vi "Output_Curve_2_2400.vi"(0 "File Path":path, 1 "V_DS Start":dbl=-0.7 format="%#.3g", 2 "V_DS Finish":dbl=3.0 format="%#.3g", 3 "V_DS Step Size":dbl=0.1 format="%#.3g", 4 "Preread delay (ms)":dbl=5000.0 format="%.2f", 5 "Delay between \naverages (ms)":dbl=200.0 format="%#.3f", 6 "Keithley 237 GPIB address":string="17", 7 "Software Averages":i16=5, 8 "VISA resource name":refnum<visa-resource-name>="GPIB0::24::INSTR", 9 "First bias settle (ms)":dbl=2000.0 format="%#.2f", 10 "V_G":dbl=0.1 format="%#_13g", 11 "Current Compliance\nLimit (A) Ke2400":dbl=0.1 format="%#.3e", 12 "Dimensions":T1(ring), 17 "Voltage Compliance Limit 237 (V)":dbl=10.0 format="%#.3f", 18 "Current Compliance\nLimit 237 (A)":dbl=0.1 format="%#.3f") -> ()   [LabVIEW 2018]
uses:
  <vilib>/Utility/file.llb/Write Delimited Spreadsheet (string).vi
  Instance           1 16Saved   JV curve .vi
  <instrlib>/Keithley 24XX/Public/Data/Read (Single Point).vi
  <vilib>/Analysis/NI_AALBase.lvlib
  <instrlib>/Keithley 24XX/Keithley 24XX.lvlib
panel:
  in  "2401":refnum<visa-resource-name>="GPIB0::22::INSTR"
  out "Keithley 2400":cluster{dbl[], dbl[]}(graph)={[-2.0, -1.9, -1.8, -1.7, -1.6, -1.5], [-6.6965744e-11, -6.7804984e-11, -6.685451799999999e-11, -6.6450076e-11, -6.5125542e-11, -6.7339852e-11]}
  out "I_G":dbl=-6.642986e-11 format="%.2e"
  in  "Autozero?":u16(ring) items=["On", "Off", "Once"]
  in  "Measurement Speed (1 PLC)":dbl=1.0 format="%.2g"
  in  "Manual Range (Max I)":dbl=1.0
  in  "Enable Meas Auto Range":bool=TRUE
  in  "Source Mode":u16(ring) items=["Voltage", "Current"]
  in  "Return Sweep?":bool
  out "I_DS":dbl=-1.38e-12 format="%.2e"
  out "Outputfile":path=path "C:/DATA/Mark Ziffer/test10"
  in  "Abort Scan":bool=TRUE
  out "V_DS":dbl=-1.5 format="%#.2f"
  out "Keithley 237":cluster{dbl[], dbl[]}(graph)={[-2.0, -1.9, -1.8, -1.7, -1.6, -1.5], [-6.720000000000001e-13, -2.18e-13, -2.7599999999999993e-13, -8.999999999999998e-14, -1.3999999999999998e-13, -1.3800000000000002e-13]}
  # "Output Curve\nbased on  EL_photocurrent_JV.vi for controlling 2 Ketthleys\n\n9/2017 MZ"
  # "Software Settings"
  # "Ke237 Settings"
  # "Ke2400 Settings"
  # "Notes for IV Scan\n\n2010.07.06 - add absolute value plotter to look at log-scale current\n2010.01.07 - Modified file headers for distinguihing when imported to Igor Pro - the prefix of each header will be the file name.\n2009.01.15 - I updated the code to run on the VISA driver convention. I also modified the file saving and the option to set the\n                      graph display.\n2008.12.01 - I fixed an issue with calculations of J. It was mis-wired to divide current by wavelength, rather than active area.  BM\n\n=========================\nI added the functionality to calculate the fill factor, rectification ratio, short circuit current density, and open circuit voltage. \nAdditionally, current density (mA/cm^2) is reported in the plot window and column B of the data file, and the current (A) has been \nmoved to column C. Open circuit voltage is linearly interpolated. The max power point (mpp) for calculating fill factor is taken as \nthe data point with the highest I-V product, so this makes it only as accurate as your voltage step size, but should be fine for a decent \ndevice on the 50 mV default step size.\n\nIf you know how to use the previous versions of IV scan, \nmake sure you set these parameters before you scan:\n1) Recftification Ratio Bias - this is the +/- bias value you wish to record a rectification ratio at.\n2) Effective Area - this is the area in cm^2 of the diode mask (photoactive area) when measuring under illumination or the measured \n     area of the electrode overlap when measured in dark (regular active area).\n3) Do you want to record a separate data file for the calculated characteristics? If so, make sure the switch is on.\n\nAs of today, I couldn't figure out how to append the computed characteristics to the I-V file without experiencing formating issues, so\nI opted to just create a separate file if you want to save that info. Feel free to fix this if you know how. Check tab 3 > tab 2 > tab 9 in the\nblock diagram.\n\n2008-04-15\nB MacLeod"
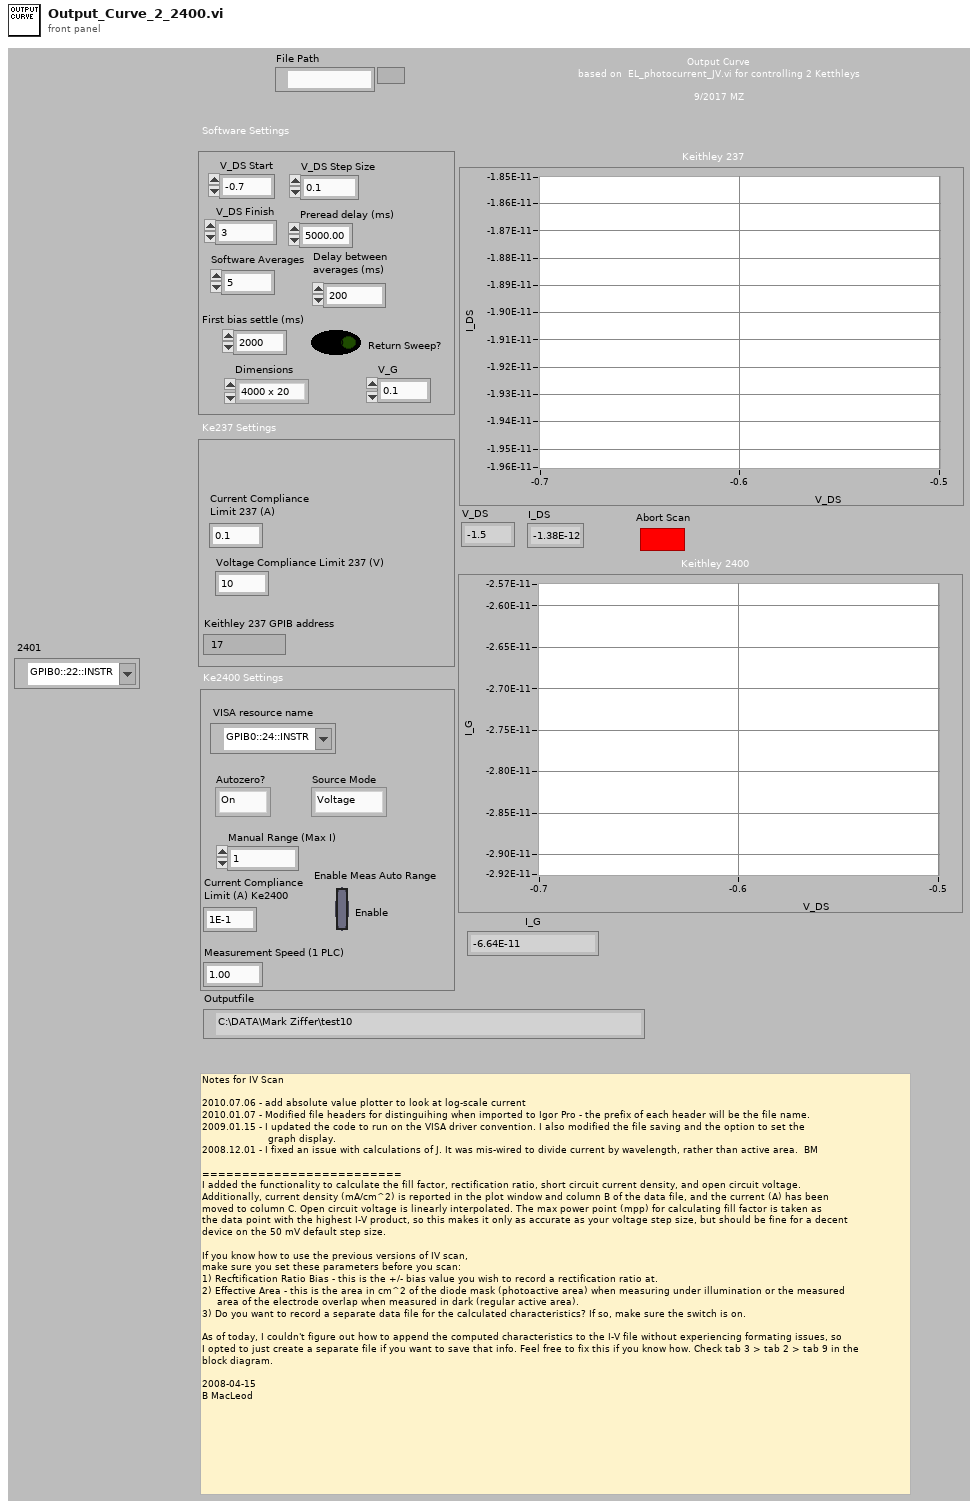
[diagram p1: front panel]
types:
  T1 = enum16{"4000 x 20", "2000 x 20", "1000 x 20", "800 x 20", "400 x 20", "200 x 20", "100 x 20"}
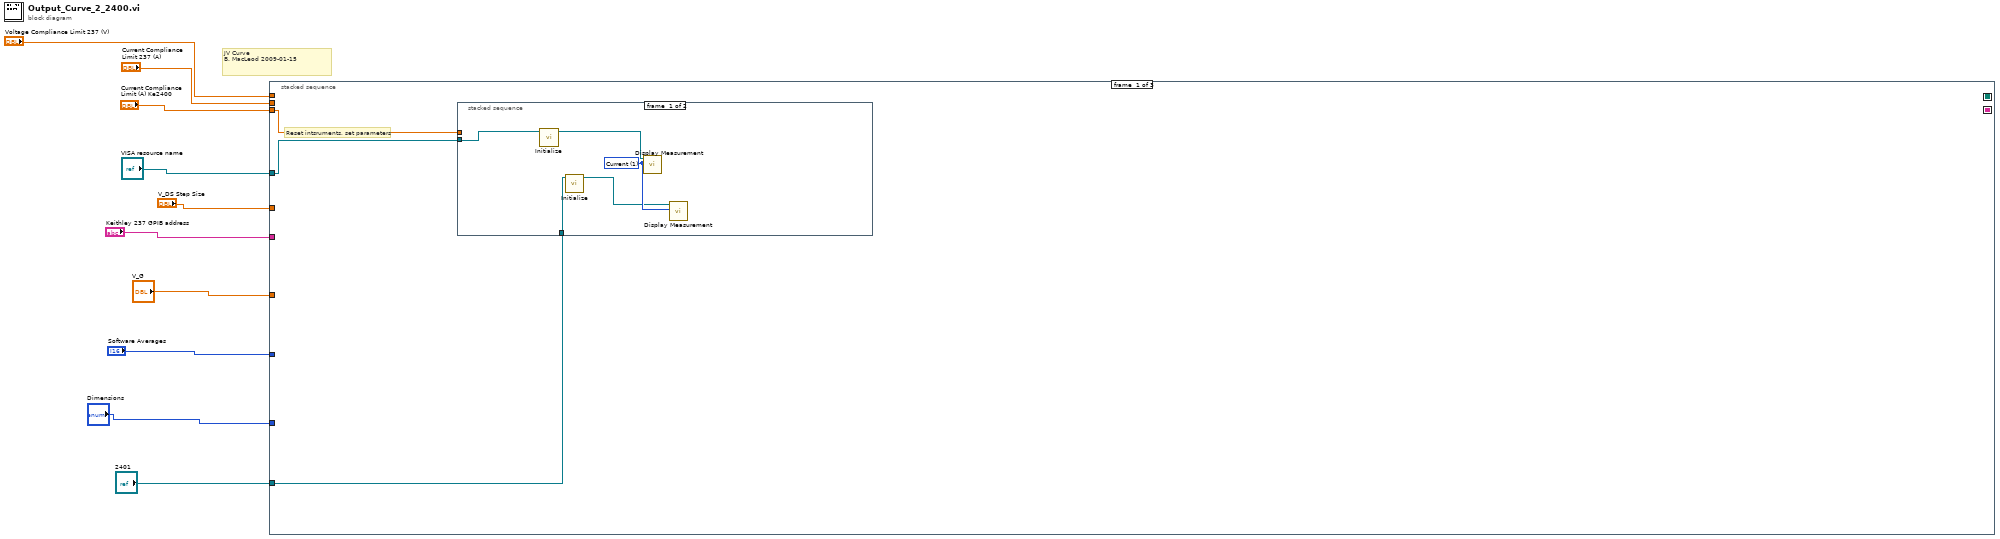
[diagram p0: block diagram]
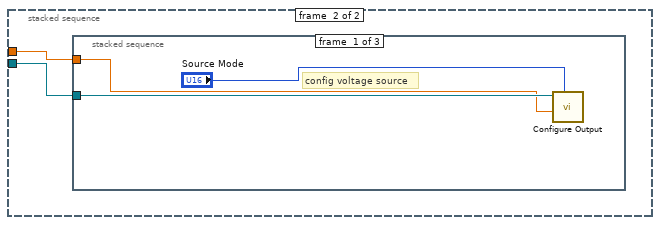
[diagram p2: hidden frame]
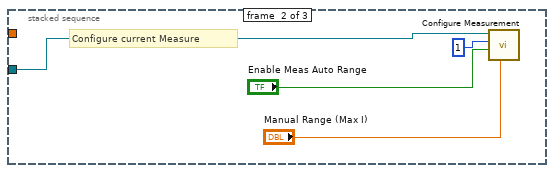
[diagram p3: hidden frame]
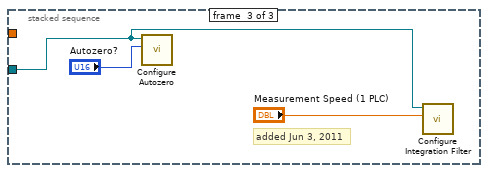
[diagram p4: hidden frame]
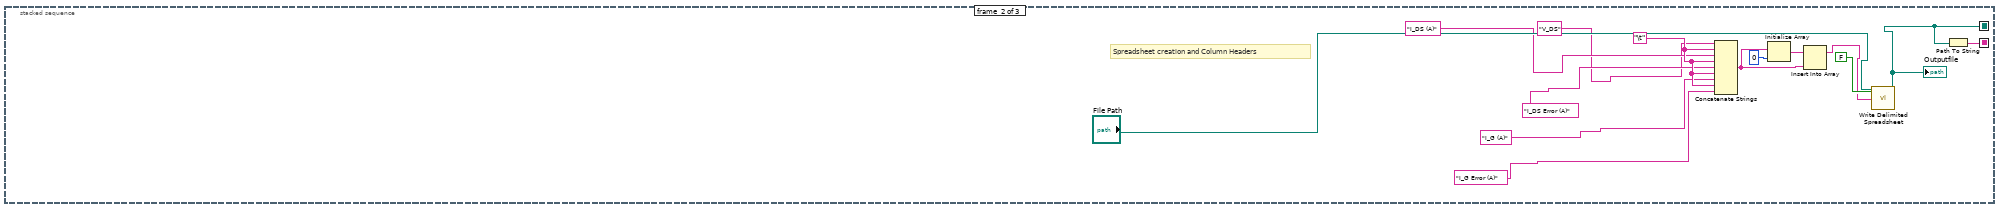
[diagram p5: hidden frame]
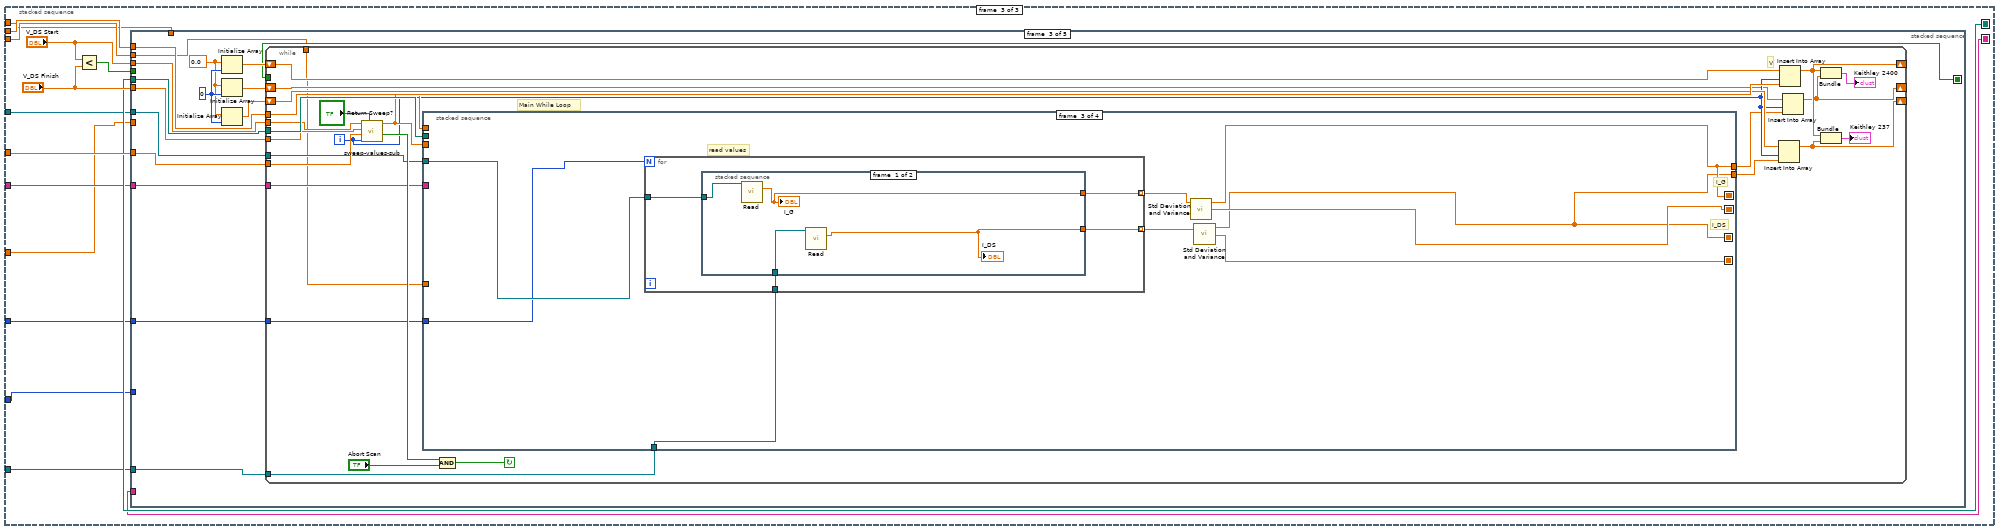
[diagram p6: hidden frame]
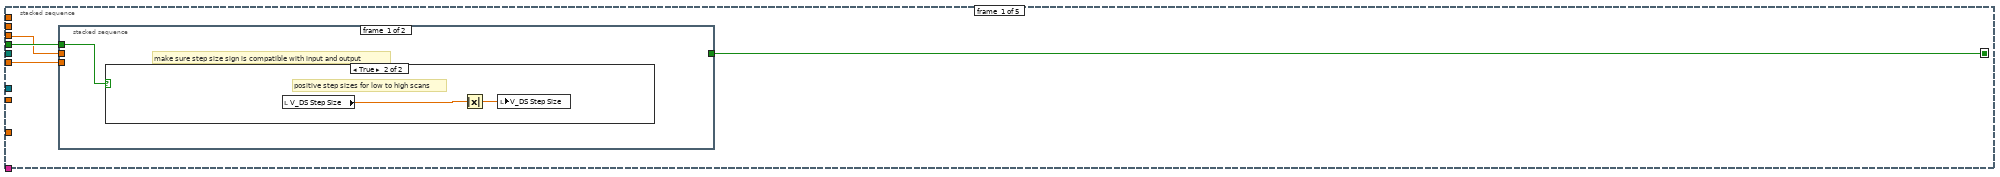
[diagram p7: hidden frame]
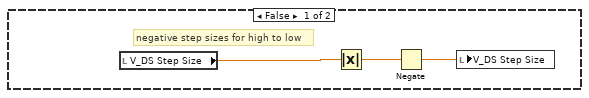
[diagram p8: hidden frame]
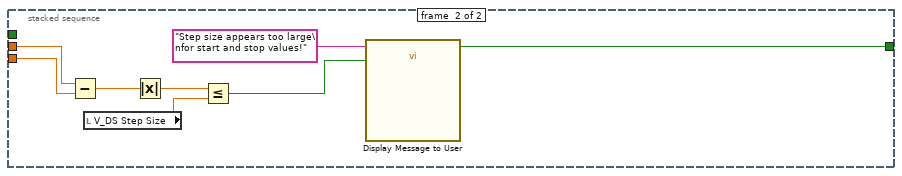
[diagram p9: hidden frame]
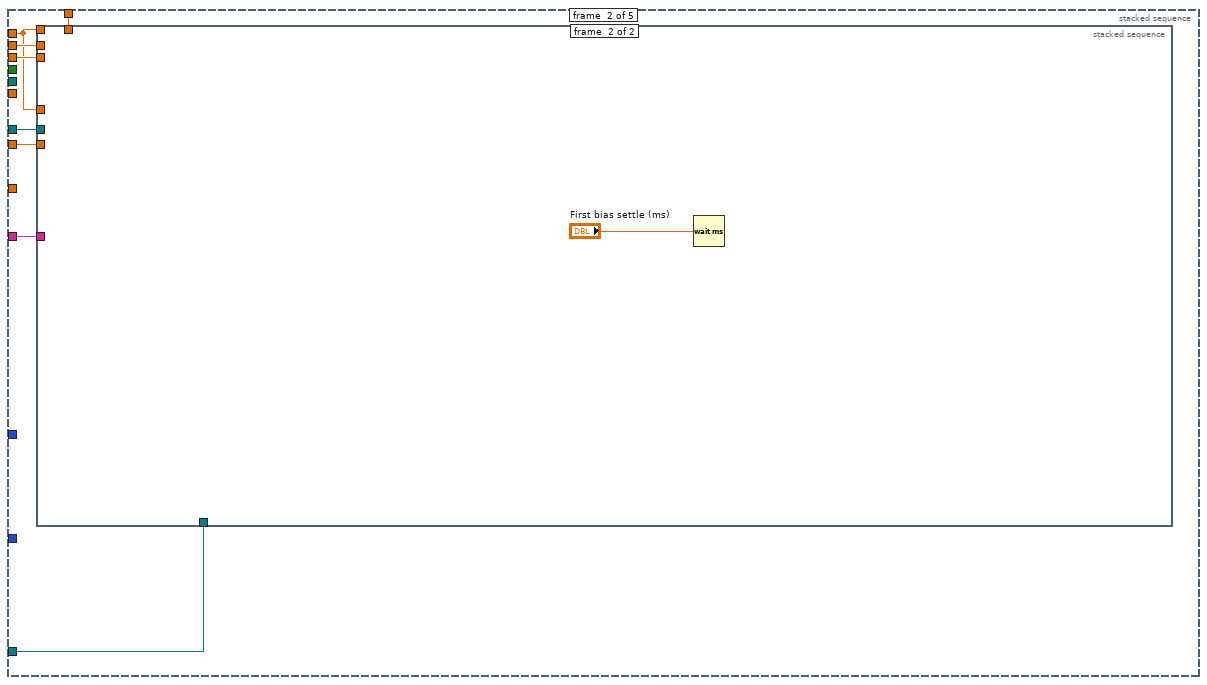
[diagram p10: hidden frame]
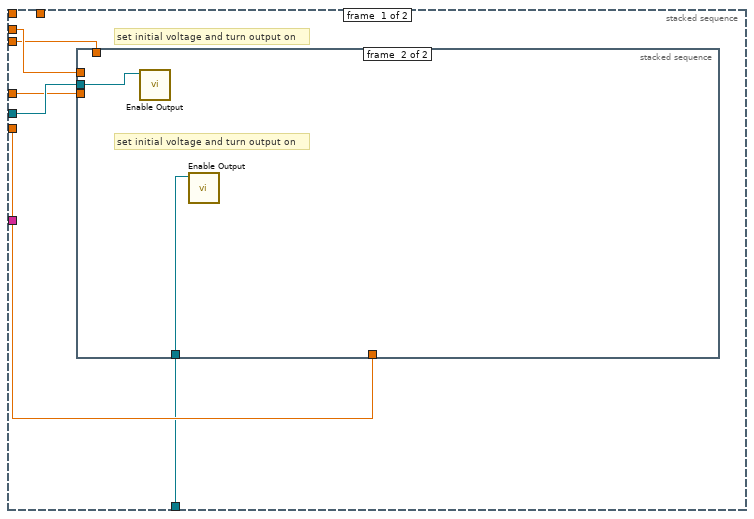
[diagram p11: hidden frame]
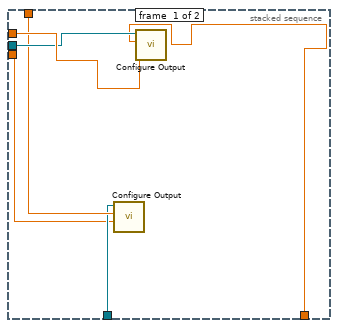
[diagram p12: hidden frame]
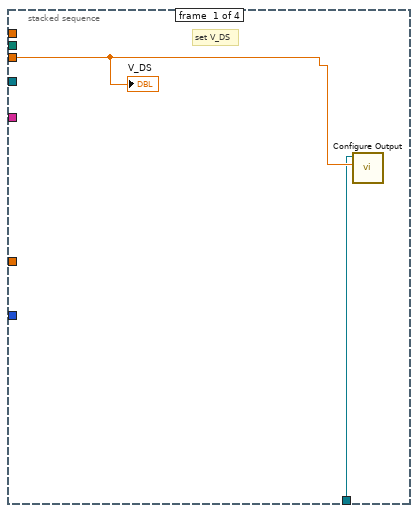
[diagram p13: hidden frame]
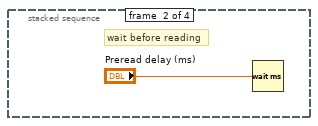
[diagram p14: hidden frame]
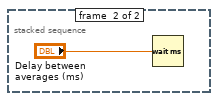
[diagram p15: hidden frame]
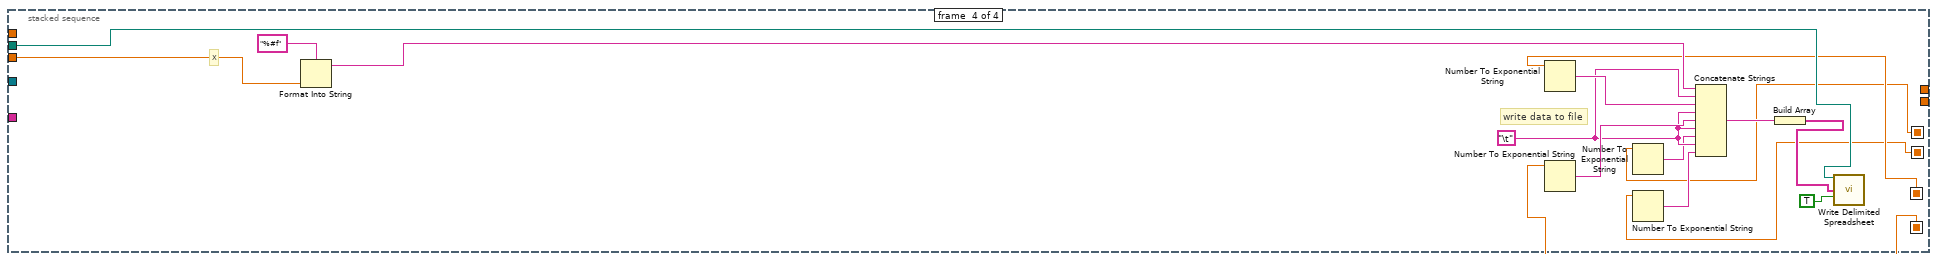
[diagram p16: hidden frame]
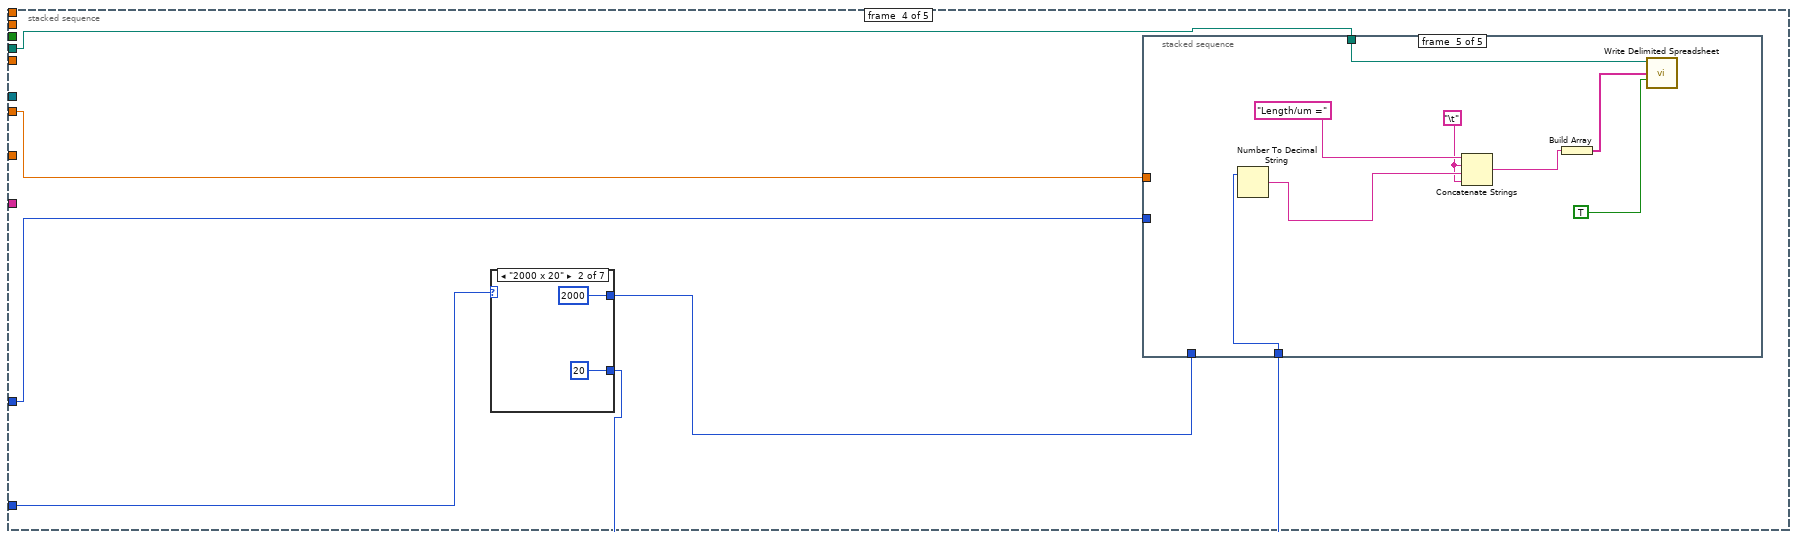
[diagram p17: hidden frame]
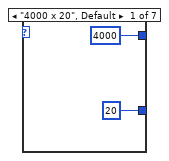
[diagram p18: hidden frame]
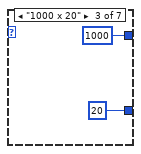
[diagram p19: hidden frame]
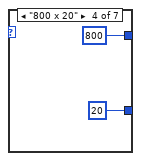
[diagram p20: hidden frame]
diagram:
  # "JV Curve\nB. MacLeod 2009-01-15"
  n1 = stacked-sequence {
    seq-local: [_ w37 _] -> [_ _ w55]
    seq-local: [_ w44 _] -> [_ _ w54]
    tunnel: "V_DS Step Size" -> [_ _ w56]
    tunnel: "Current Compliance\nLimit 237 (A)" -> [_ _ w53]
    tunnel: "Voltage Compliance Limit 237 (V)" -> [_ _ w49]
    tunnel: "Keithley 237 GPIB address" -> [_ _ w52]
    tunnel: "VISA resource name" -> [w13 _ w51]
    tunnel: "Current Compliance\nLimit (A) Ke2400" -> [w12 _ w50]
    tunnel: "V_G" -> [_ _ w48]
    tunnel: "Software Averages" -> [_ _ w47]
    tunnel: "Dimensions" -> [_ _ w46]
    tunnel: "2401" -> [w11 _ w45]
    frame #0 {
      # "Reset intsruments, set parameters"
      n2 = stacked-sequence {
        tunnel: w13 -> [w18 w20]
        tunnel: w12 -> [_ w19]
        tunnel: w11 -> [w14 _]
        frame #0 {
          w16 = u16 1 items=["Voltage", "Current", "Resistance"] ("Displayed Measurement (0: Voltage)")
          n3 = call <instrlib>:"Initialize.vi"("VISA resource name"=w18) -> ("VISA resource name out"=w17:refnum<visa-resource-name>)  [unwired: 9 in, 1 out]
          n4 = call <instrlib>:"Initialize.vi"("VISA resource name"=w14) -> ("VISA resource name out"=w15:refnum<visa-resource-name>)  [unwired: 9 in, 1 out]
          n5 = call <instrlib>:"Display Measurement.vi"("Displayed Measurement (0: Voltage)"=w16, "VISA resource name"=w17) -> ()  [unwired: 8 in, 2 out]
          n6 = call <instrlib>:"Display Measurement.vi"("Displayed Measurement (0: Voltage)"=w16, "VISA resource name"=w15) -> ()  [unwired: 8 in, 2 out]
        }
        frame #1 {
          n7 = stacked-sequence {
            tunnel: w20 -> [w22 w24 w28]
            tunnel: w19 -> [w21 _ _]
            frame #0 {
              # "config voltage source"
              n8 = call <instrlib>:"Configure Output.vi"("Source Mode  (0: Voltage)"="Source Mode", "Compliance  Level (0.1)"=w21, "VISA resource name"=w22) -> ()  [unwired: 3 in, 6 out]
            }
            frame #1 {
              # "Configure current Measure"
              n9 = call <instrlib>:"Configure Measurement.vi"("Manual Range (1.0)"="Manual Range (Max I)", "Enable Auto Range (T:Enable)"="Enable Meas Auto Range", "Function (0: Volts)"=1, "VISA resource name"=w24) -> ()  [unwired: 1 in, 7 out]
            }
            frame #2 {
              # "added Jun 3, 2011"
              n10 = call <instrlib>:"Configure Autozero.vi"("Autozero  (0: On)"="Autozero?", "VISA resource name"=w28) -> ()  [unwired: 1 in, 9 out]
              n11 = call <instrlib>:"Configure Integration Filter.vi"("Measurement Speed (1 PLC)"="Measurement Speed (1 PLC)", "VISA resource name"=w28) -> ()  [unwired: 8 in, 2 out]
            }
          }
        }
      }
    }
    frame #1 {
      w40 = "\t"
      # "Spreadsheet creation and Column Headers"
      n12 = Concatenate Strings("V_DS", w40, "I_DS (A)", w40, "I_DS Error (A)", w40, "I_G (A)", w40, "I_G Error (A)" ("string")) -> (w42:string)
      n13 = Initialize Array(w42, 0 ("dimension size")) -> (w41:string[])
      n14 = Insert Into Array(array=w41, new element=w42) -> (w38:string[])  [unwired: 1 in]
      n15 = call-poly <vilib>:"Write Delimited Spreadsheet.vi"("file path (dialog if empty)"="File Path", "1D data"=w38, "transpose? (no:F)"=FALSE ("append to file? (new file:F)")) -> ("new file path (Not A Path if cancelled)"=w37:path)  [unwired: 11 in, 1 out]
      "Outputfile" <- w37
      n16 = Path To String(path=w37) -> (string=w44:string)
    }
    frame #2 {
      n17 = Less?(x="V_DS Start", y="V_DS Finish") -> (x < y?=w57:bool)
      n18 = stacked-sequence {
        seq-local: [w60 _ _ _ _] -> [_ _ w109 _ _]
        tunnel: w57 -> [w63 _ _ _ _]
        tunnel: "V_DS Start" -> [w62 w81 w115 _ _]
        tunnel: "V_DS Finish" -> [w61 _ w116 _ _]
        tunnel: w56 -> [_ _ w114 _ _]
        tunnel: w55 -> [_ _ w113 w183 _]
        tunnel: w54 -> [_ _ _ _ _]
        tunnel: w53 -> [_ w78 w110 _ _]
        tunnel: w52 -> [_ w85 w108 _ w240]
        tunnel: w51 -> [_ w83 w107 _ w239]
        tunnel: w50 -> [_ w84 w103 _ _]
        tunnel: w49 -> [_ w82 _ _ _]
        tunnel: w48 -> [_ w80 _ w185 _]
        tunnel: w47 -> [_ _ w102 w184 _]
        tunnel: w46 -> [_ _ _ w182 _]
        tunnel: w45 -> [_ w79 w101 _ _]
        frame #0 {
          n19 = stacked-sequence {
            tunnel: w63 -> [w64 _]
            tunnel: w62 -> [_ w77]
            tunnel: w61 -> [_ w76]
            tunnel: [_ w70] -> w60
            frame #0 {
              # "make sure step size sign is compatible with input and output"
              n20 = case shown="True" w64 {
                frame False {
                  # "negative step sizes for high to low"
                  n21 = local read "V_DS Step Size"() -> (w67:dbl)
                  n22 = Absolute Value(x=w67) -> (abs(x)=w66:dbl)
                  n23 = Negate(x=w66) -> (-x=w65:dbl)
                  n24 = local write "V_DS Step Size"(w65) -> ()
                }
                frame True {
                  # "positive step sizes for low to high scans"
                  n25 = local read "V_DS Step Size"() -> (w69:dbl)
                  n26 = Absolute Value(x=w69) -> (abs(x)=w68:dbl)
                  n27 = local write "V_DS Step Size"(w68) -> ()
                }
              }
            }
            frame #1 {
              n28 = Subtract(x=w77, y=w76) -> (x-y=w75:dbl)
              n29 = local read "V_DS Step Size"() -> (w73:dbl)
              n30 = Absolute Value(x=w75) -> (abs(x)=w74:dbl)
              n31 = Less Or Equal?(x=w74, y=w73) -> (x <= y?=w71:bool)
              n32 = call "Display Message to User"("Enable"=w71, "Message"="Step size appears too large\nfor start and stop values!") -> ("OK"=w70:bool)  [unwired: 1 in, 8 out]
            }
          }
        }
        frame #1 {
          n33 = stacked-sequence {
            tunnel: w78 -> [_ _]
            tunnel: w85 -> [_ _]
            tunnel: w84 -> [w91 _]
            tunnel: w83 -> [w90 _]
            tunnel: w82 -> [_ _]
            tunnel: w81 -> [w88 _]
            tunnel: w80 -> [w89 _]
            tunnel: w79 -> [w87 _]
            tunnel: w78 -> [w86 _]
            frame #0 {
              # "set initial voltage and turn output on"
              # "set initial voltage and turn output on"
              n34 = stacked-sequence {
                tunnel: w91 -> [w97 _]
                tunnel: w90 -> [w96 w99]
                tunnel: w89 -> [w95 _]
                tunnel: w88 -> [w94 _]
                tunnel: w87 -> [w93 w98]
                tunnel: w86 -> [w92 _]
                frame #0 {
                  n35 = call <instrlib>:"Configure Output.vi"("Compliance  Level (0.1)"=w92, "Output Level (0)"=w94, "VISA resource name"=w93) -> ()  [unwired: 3 in, 6 out]
                  n36 = call <instrlib>:"Configure Output.vi"("Compliance  Level (0.1)"=w97, "Output Level (0)"=w95, "VISA resource name"=w96) -> ()  [unwired: 3 in, 6 out]
                }
                frame #1 {
                  n37 = call <instrlib>:"Enable Output.vi"("VISA resource name"=w99) -> ()  [unwired: 2 in, 9 out]
                  n38 = call <instrlib>:"Enable Output.vi"("VISA resource name"=w98) -> ()  [unwired: 2 in, 9 out]
                }
              }
            }
            frame #1 {
              n39 = Wait (ms)(milliseconds to wait="First bias settle (ms)") -> ()  [unwired: 1 out]
            }
          }
        }
        frame #2 {
          w106 = 0
          w105 = 0.0
          n40 = Initialize Array(w105, w106) -> (w112:dbl[])
          n41 = Initialize Array(w105, w106) -> (w104:dbl[])
          n42 = Initialize Array(w105, w106) -> (w111:dbl[])
          n43 = while {
            shift-left: w111 -> [w138]
            shift-right: [w126] -> _
            shift-left: w112 -> [w139]
            shift-right: [w129] -> _
            tunnel: w113 -> [w141]
            tunnel: w114 -> [w137]
            tunnel: w115 -> [w136]
            tunnel: w116 -> [w135]
            tunnel: w110 -> [w133]
            tunnel: w109 -> [_]
            shift-right: [w125] -> _
            shift-left: w104 -> [w121]
            tunnel: w108 -> [w124]
            tunnel: w107 -> [w123]
            tunnel: w103 -> [w119]
            tunnel: w102 -> [w118]
            tunnel: w101 -> [w117]
            i -> [w127]
            stop <- w131 continue-if-true
            # "Main While Loop"
            # "V"
            n44 = call "sweep-values-sub.vi"("Forward/Reverse"="Return Sweep?", "Point Number"=w127, "Step Size"=w137, "Sweep Stop"=w135, "Sweep Start"=w136) -> ("Active"=w132:bool, "Output"=w140:dbl)  [unwired: 2 out]
            n45 = stacked-sequence {
              seq-local: [_ _ w154 _] -> [_ _ _ w166]
              seq-local: [_ _ w149 _] -> [_ _ _ w167]
              seq-local: [_ _ w151 _] -> [_ _ _ w165]
              seq-local: [_ _ w150 _] -> [_ _ _ w164]
              tunnel: [_ _ w149 _] -> w128
              tunnel: w140 -> [w144 _ _ w178]
              tunnel: w141 -> [_ _ _ w169]
              tunnel: w133 -> [_ _ _ _]
              tunnel: w124 -> [_ _ _ _]
              tunnel: w123 -> [_ _ w152 _]
              tunnel: [_ _ w151 _] -> w122
              tunnel: w119 -> [_ _ _ _]
              tunnel: w118 -> [_ _ w148 _]
              tunnel: w117 -> [w143 _ w146 _]
              frame #0 {
                # "set V_DS"
                n46 = call <instrlib>:"Configure Output.vi"("Output Level (0)"=w144, "VISA resource name"=w143) -> ()  [unwired: 8 in, 2 out]
                "V_DS" <- w144
              }
              frame #1 {
                # "wait before reading"
                n47 = Wait (ms)(milliseconds to wait="Preread delay (ms)") -> ()  [unwired: 1 out]
              }
              frame #2 {
                # "I_DS"
                # "I_G"
                # "read values"
                n48 = for {
                  N: w148 -> [_]
                  tunnel: [w158] -> w153 mode=indexing
                  tunnel: w152 -> [w157]
                  tunnel: [w156] -> w147 mode=indexing
                  tunnel: w146 -> [w155]
                  n49 = stacked-sequence {
                    tunnel: [w159 _] -> w158
                    tunnel: w157 -> [w162 _]
                    tunnel: [w161 _] -> w156
                    tunnel: w155 -> [w160 _]
                    frame #0 {
                      n50 = call-poly <instrlib>:"Read.vi"("VISA resource name"=w162) -> ("Current"=w161:sgl)  [unwired: 8 in, 6 out]
                      "I_G" <- w161
                      n51 = call-poly <instrlib>:"Read.vi"("VISA resource name"=w160) -> ("Current"=w159:sgl)  [unwired: 8 in, 6 out]
                      "I_DS" <- w159
                    }
                    frame #1 {
                      n52 = Wait (ms)(milliseconds to wait="Delay between \naverages (ms)") -> ()  [unwired: 1 out]
                    }
                  }
                }
                n53 = call <vilib>:"Std Deviation and Variance.vi"("X"=w147) -> ("mean"=w151:dbl, "standard deviation"=w150:dbl)  [unwired: 1 in, 1 out]
                n54 = call <vilib>:"Std Deviation and Variance.vi"("X"=w153) -> ("mean"=w149:dbl, "standard deviation"=w154:dbl)  [unwired: 1 in, 1 out]
              }
              frame #3 {
                w173 = "\t"
                # "write data to file"
                # "X"
                n55 = Format Into String(format string="%#f", w178) -> (resulting string=w176:string)  [unwired: 2 in, 1 out]
                n56 = Number To Exponential String(number=w167) -> (E-format string=w179:string)  [unwired: 3 out]
                n57 = Number To Exponential String(number=w166) -> (E-format string=w175:string)  [unwired: 3 out]
                n58 = Number To Exponential String(number=w165) -> (E-format string=w172:string)  [unwired: 3 out]
                n59 = Number To Exponential String(number=w164) -> (E-format string=w171:string)  [unwired: 3 out]
                n60 = Concatenate Strings(w176, w173, w179, w173, w175, w173, w172, w173, w171) -> (w174:string)
                n61 = Build Array(w174) -> (w170:string[])
                n62 = call-poly <vilib>:"Write Delimited Spreadsheet.vi"("file path (dialog if empty)"=w169, "1D data"=w170, "append to file? (new file:F)"=TRUE) -> ()  [unwired: 11 in, 2 out]
              }
            }
            n63 = Compound Arithmetic op=AND(w132, "Abort Scan") -> (w131:bool)
            n64 = Insert Into Array(array=w138, index=w127, new element=w128) -> (w126:dbl[])
            n65 = Insert Into Array(array=w139, index=w127, new element=w140) -> (w129:dbl[])
            n66 = Insert Into Array(array=w121, index=w127, new element=w122) -> (w125:dbl[])
            n67 = Bundle(w129, w125) -> (→"Keithley 2400":cluster{dbl[], dbl[]})  [unwired: 1 out]
            n68 = Bundle(w129, w126) -> (→"Keithley 237":cluster{dbl[], dbl[]})  [unwired: 1 out]
          }
        }
        frame #3 {
          n69 = case shown="\"2000 x 20\"" w182 {
            tunnel: [4000 2000 1000 800 400 200 100] -> w181
            tunnel: [20 20 20 20 20 20 20] -> w180
            frame "4000 x 20", Default {
            }
            frame "2000 x 20" {
            }
            frame "1000 x 20" {
            }
            frame "800 x 20" {
            }
            frame "400 x 20" {
            }
            frame "200 x 20" {
            }
            frame "100 x 20" {
            }
          }
          n70 = stacked-sequence {
            tunnel: w185 -> [_ w211 _ _ _]
            tunnel: w183 -> [w200 w209 w215 w223 w231]
            tunnel: w184 -> [_ _ w217 _ _]
            tunnel: w181 -> [_ _ _ w224 _]
            tunnel: w180 -> [_ _ _ _ w232]
            frame #0 {
              w205 = ""
              w204 = "\t"
              n71 = Concatenate Strings(w205, w204, w205, w204) -> (w201:string)
              n72 = Build Array(w201) -> (w203:string[])
              n73 = call-poly <vilib>:"Write Delimited Spreadsheet.vi"("file path (dialog if empty)"=w200, "1D data"=w203, "append to file? (new file:F)"=TRUE) -> ()  [unwired: 11 in, 2 out]
            }
            frame #1 {
              w212 = "\t"
              n74 = Number To Fractional String(number=w211, precision (6)=3) -> (F-format string=w210:string)  [unwired: 2 in]
              n75 = Concatenate Strings("V_G = ", w212, w210, w212) -> (w213:string)
              n76 = Build Array(w213) -> (w208:string[])
              n77 = call-poly <vilib>:"Write Delimited Spreadsheet.vi"("file path (dialog if empty)"=w209, "1D data"=w208, "append to file? (new file:F)"=TRUE) -> ()  [unwired: 11 in, 2 out]
            }
            frame #2 {
              w220 = "\t"
              n78 = Number To Decimal String(number=w217) -> (decimal integer string=w216:string)  [unwired: 1 in]
              n79 = Concatenate Strings("Number of Averages = ", w220, w216, w220) -> (w221:string)
              n80 = Build Array(w221) -> (w219:string[])
              n81 = call-poly <vilib>:"Write Delimited Spreadsheet.vi"("file path (dialog if empty)"=w215, "1D data"=w219, "append to file? (new file:F)"=TRUE) -> ()  [unwired: 11 in, 2 out]
            }
            frame #3 {
              w228 = "\t"
              n82 = Number To Decimal String(number=w224) -> (decimal integer string=w227:string)  [unwired: 1 in]
              n83 = Concatenate Strings("Width/um =", w228, w227, w228) -> (w226:string)
              n84 = Build Array(w226) -> (w225:string[])
              n85 = call-poly <vilib>:"Write Delimited Spreadsheet.vi"("file path (dialog if empty)"=w223, "1D data"=w225, "append to file? (new file:F)"=TRUE) -> ()  [unwired: 11 in, 2 out]
            }
            frame #4 {
              w233 = "\t"
              n86 = Number To Decimal String(number=w232) -> (decimal integer string=w236:string)  [unwired: 1 in]
              n87 = Concatenate Strings("Length/um =", w233, w236, w233) -> (w237:string)
              n88 = Build Array(w237) -> (w238:string[])
              n89 = call-poly <vilib>:"Write Delimited Spreadsheet.vi"("file path (dialog if empty)"=w231, "1D data"=w238, "append to file? (new file:F)"=TRUE) -> ()  [unwired: 11 in, 2 out]
            }
          }
        }
        frame #4 {
          # "reset instrument at end of sweep"
          n90 = call <instrlib>:"Reset.vi"("VISA resource name"=w239) -> ()  [unwired: 9 in, 2 out]
          n91 = call <userlib>:"Keith 237 Reset.vi"("GPIB address"=w240) -> ()  [unwired: 1 in, 1 out]
        }
      }
    }
  }
